vi "Clear Buffers.vi"(8 "error in":errorcluster, 11 "Serial IO in":refnum<class "Serial IO.lvclass">) -> (0 "error out":errorcluster, 3 "Serial IO out":refnum<class "Serial IO.lvclass">)   [LabVIEW 2015, in "Serial IO.lvclass"]
uses:
  Serial IO.lvclass
  Serial IO.lvclass/Serial IO.ctl
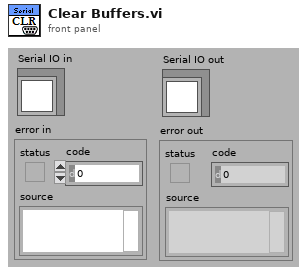
[diagram p1: front panel]
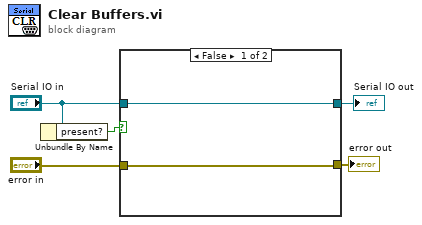
[diagram p0: block diagram]
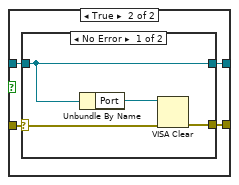
[diagram p2: hidden frame]
diagram:
  n1 = Unbundle By Name("Serial IO in") -> ("present?"=w1:bool)
  n2 = case shown="False" w1 {
    tunnel: "error in" -> [w6 w11]
    tunnel: [w6 w10] -> w4
    tunnel: "Serial IO in" -> [w7 w9]
    tunnel: [w7 w8] -> w3
    frame False {
    }
    frame True {
      n3 = case shown="No Error" w11 {
        selector: w11 -> [w14 w17]
        tunnel: [w13 w17] -> w10
        tunnel: [w12 w16] -> w8
        tunnel: w9 -> [w12 w16]
        frame No Error {
          n4 = Unbundle By Name(w12) -> ("Port"=w15:refnum<visa-resource-name>)
          n5 = VISA Clear(VISA resource name=w15, error in (no error)=w14) -> (error out=w13:errorcluster)  [unwired: 1 out]
        }
        frame Error {
        }
      }
    }
  }
  "error out" <- w4
  "Serial IO out" <- w3
